vi "OnDrop.vi"(0 "XRef":T13, 1 "State In":T1) -> (14 "Reply":T11, 15 "Fatal Error Out":T10, 16 "State Out":T1)   [LabVIEW 2020, in "FlexBlock.xnode"]
uses:
  FlexBlock.xnode
  <vilib>/XNodeSupport/XNodeXNodeRef.ctl
  State.ctl
  FlexBlocks/Type Descriptor.ctl
  FlexBlocks/Terminal Direction.ctl
  FlexBlocks/Value Mode.ctl
  FlexBlocks/Terminal State.ctl
  FlexBlocks/Special Terminal.ctl
  FlexBlocks/Errors.ctl
  <vilib>/picture/picture.llb/imagedata.ctl
  FlexBlocks/Calculated Sizes.ctl
  <vilib>/XNodeSupport/XNodeStringArray.ctl
  <vilib>/XNodeSupport/XNodeString.ctl
  <vilib>/XNodeSupport/XNodeErrorCluster.ctl
  <vilib>/XNodeSupport/NI_XNodeSupport.lvlib
  FlexBlocks/FlexBlocks.lvlib
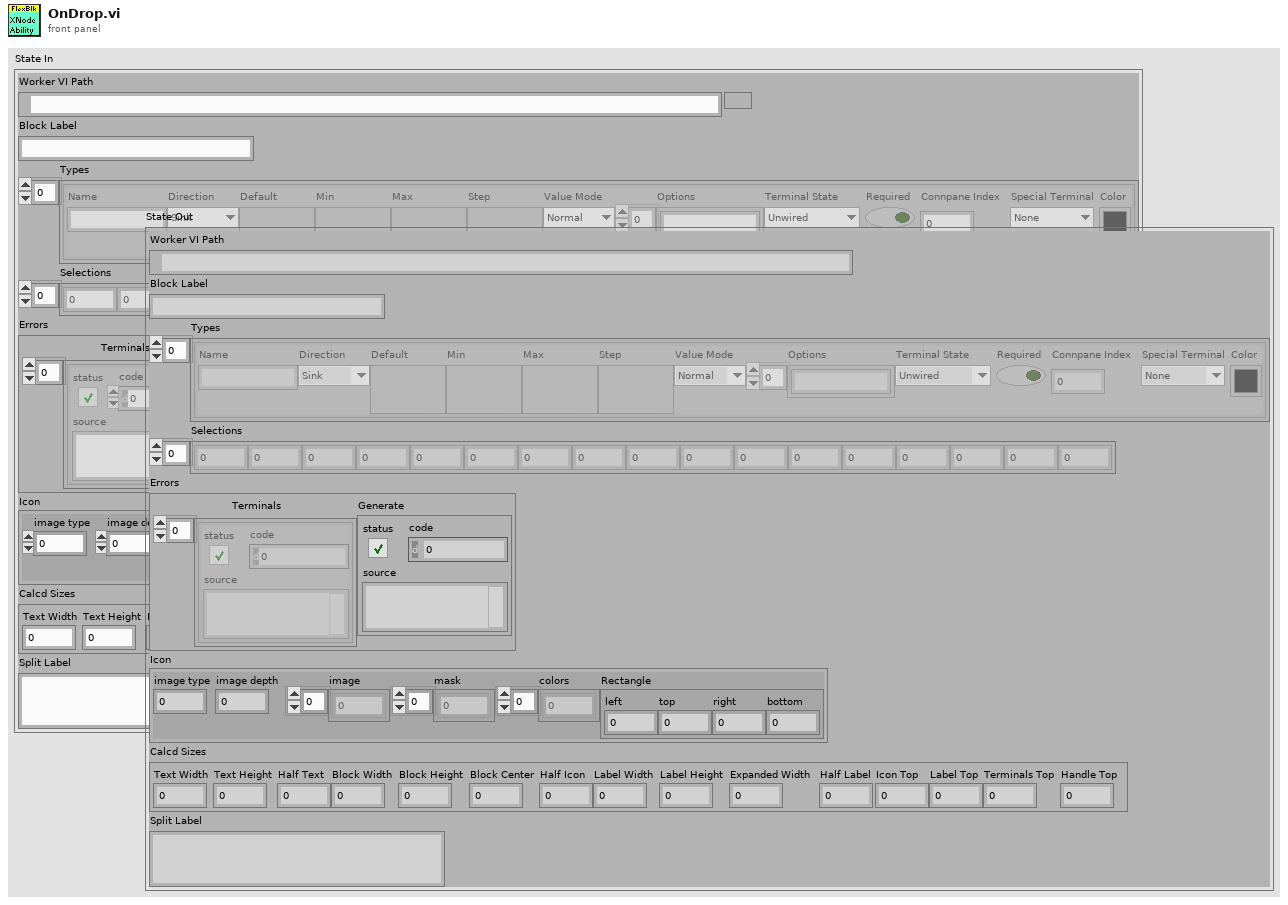
[diagram p1: front panel]
types:
  T1 = typedef "FlexBlock.xnode/State.ctl" = cluster{"Worker VI Path":path, "Block Label":string, "Types":T2[], "Selections":i32[], "Errors":T7, "Icon":T8, "Calcd Sizes":T9, "Split Label":string}
  T2 = typedef "FlexBlocks.lvlib/Type Descriptor.ctl" = cluster{"Name":string, "Direction":T3, "Default":variant, "Min":variant, "Max":variant, "Step":variant, "Value Mode":T4, "Options":string[], "Terminal State":T5, "Required":bool, "Connpane Index":i32, "Special Terminal":T6, "Color":u32}
  T3 = typedef "FlexBlocks.lvlib/Terminal Direction.ctl" = enum16{"Sink", "Source"}
  T4 = typedef "FlexBlocks.lvlib/Value Mode.ctl" = enum16{"Normal", "Range", "Select"}
  T5 = typedef "FlexBlocks.lvlib/Terminal State.ctl" = enum16{"Unwired", "BadType", "BadRef", "Channel", "Value", "Control Ref"}
  T6 = typedef "FlexBlocks.lvlib/Special Terminal.ctl" = enum16{"None", "Action", "Init", "Tag", "State in", "State out", "Error"}
  T7 = typedef "FlexBlocks.lvlib/Errors.ctl" = cluster{"Terminals":errorcluster[], "Generate":errorcluster}
  T8 = typedef "imagedata.ctl" = cluster{"image type":i32, "image depth":i32, "image":u8[], "mask":u8[], "colors":u32[], "Rectangle":cluster{"left":i16, "top":i16, "right":i16, "bottom":i16}}
  T9 = typedef "FlexBlocks.lvlib/Calculated Sizes.ctl" = cluster{"Text Width":i32, "Text Height":i32, "Half Text":i32, "Block Width":i32, "Block Height":i32, "Block Center":i32, "Half Icon":i32, "Label Width":i32, "Label Height":i32, "Expanded Width":i32, "Half Label":i32, "Icon Top":i32, "Label Top":i32, "Terminals Top":i32, "Handle Top":i32}
  T10 = typedef "NI_XNodeSupport.lvlib/XNodeErrorCluster.ctl" = errorcluster
  T11 = typedef "NI_XNodeSupport.lvlib/XNodeStringArray.ctl" = T12[]
  T12 = typedef "NI_XNodeSupport.lvlib/XNodeString.ctl" = string
  T13 = typedef "NI_XNodeSupport.lvlib/XNodeXNodeRef.ctl" = refnum<vi>
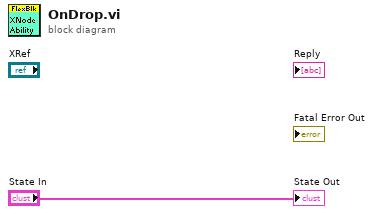
[diagram p0: block diagram]
diagram:
  "State Out" <- "State In"
